vi "Set First Values.vi"(6 "PAYLOAD":u32[](array[numeric])=[0, 0, 0, 0, 0, 0, 0, 0, 0, 0, 0, 0, 0, 0, 0, 0, 0, 0, 0, 0, 0, 0, 0, 0, 0, 0, 0, 0, 0, 0, 0, 0, 0, 0, 0, 0, 0, 0, 0, 0, 0, 0, 0, 0, 0, 0, 0, 0, 0, 0, 0, 0, 0, 0, 0, 0, 0, 0, 0, 0, 0, 0, 0, 0] format="%x", 7 "TYPE":T1 items=["CAN Data"=0, "CAN Remote"=1, "CAN Bus Error"=2, "CAN 2.0 Data"=8, "CAN FD Data"=16, "CAN FD+BRS Data"=24, "J1939 Data"=192, "Delay"=224, "Log Trigger"=225, "Start Trigger"=226], 8 "error":errorcluster, 9 "DLC":u32 format="%x", 10 "IDENTIFIER":u32 format="%x", 11 "gRPC ID In":T2) -> (0 "error out":errorcluster, 3 "gRPC ID Out":T2)   [LabVIEW 2025]
uses:
  <vilib>/gRPC/LabVIEW gRPC Library/Shared/grpcId.ctl
  OOB gRPC Client/RPC Messages/hwval_GenericRequest.ctl
  OOB gRPC Client/OOB gRPC Client.lvlib
  <vilib>/gRPC/LabVIEW gRPC Library/grpc-lvsupport-release.lvlib
  XNET Frame Type CAN.ctl
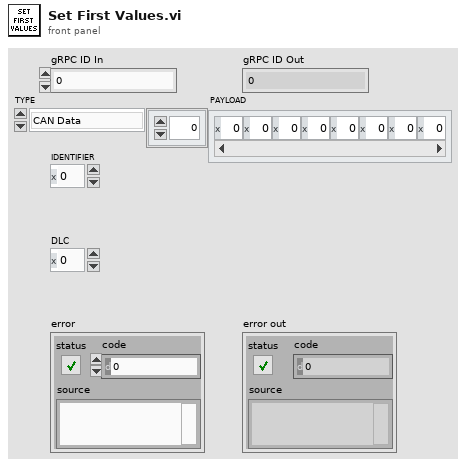
[diagram p1: front panel]
types:
  T1 = typedef "XNET Frame Type CAN.ctl" = u32
  T2 = typedef "grpc-lvsupport-release.lvlib/grpcId.ctl" = u64
  T3 = typedef "OOB gRPC Client.lvlib/hwval_GenericRequest.ctl" = cluster{"Command":string, "Payload":u8[]}
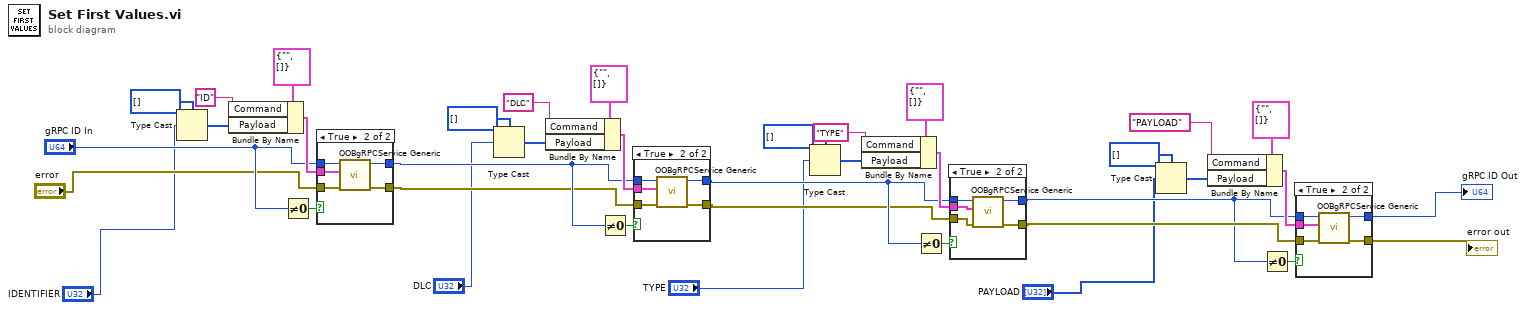
[diagram p0: block diagram]
diagram:
  n1 = Type Cast(type=u8[] [] ("Payload"), x="IDENTIFIER") -> (*(type *) &x=w35:u8[])
  n2 = Bundle By Name(cluster=T3 {"Command"="", "Payload"=[]} ("hwval_GenericRequest"), "Command"="ID", "Payload"=w35) -> (w34:T3)
  n3 = Not Equal To 0?(x="gRPC ID In") -> (x != 0?=w33:bool)
  n4 = case shown="True" w33 {
    tunnel: [w40 w42] -> w23
    tunnel: [w39 w41] -> w22
    tunnel: "gRPC ID In" -> [w40 w45]
    tunnel: "error" -> [w39 w44]
    tunnel: w34 -> [_ w43]
    frame False {
    }
    frame True {
      n5 = call "OOBgRPCService Generic.vi"("error in"=w44, "Request Data"=w43, "gRPC ID"=w45) -> ("error out"=w41:errorcluster, "gRPC ID out"=w42:T2)  [unwired: 6 in, 1 out]
    }
  }
  n6 = Type Cast(type=u8[] [] ("Payload"), x="DLC") -> (*(type *) &x=w26:u8[])
  n7 = Bundle By Name(cluster=T3 {"Command"="", "Payload"=[]} ("hwval_GenericRequest"), "Command"="DLC", "Payload"=w26) -> (w25:T3)
  n8 = Not Equal To 0?(x=w23) -> (x != 0?=w24:bool)
  n9 = case shown="True" w24 {
    tunnel: [w47 w49] -> w14
    tunnel: [w46 w48] -> w13
    tunnel: w23 -> [w47 w52]
    tunnel: w22 -> [w46 w51]
    tunnel: w25 -> [_ w50]
    frame False {
    }
    frame True {
      n10 = call "OOBgRPCService Generic.vi"("error in"=w51, "Request Data"=w50, "gRPC ID"=w52) -> ("error out"=w48:errorcluster, "gRPC ID out"=w49:T2)  [unwired: 6 in, 1 out]
    }
  }
  n11 = Type Cast(type=u8[] [] ("Payload"), x="TYPE") -> (*(type *) &x=w17:u8[])
  n12 = Bundle By Name(cluster=T3 {"Command"="", "Payload"=[]} ("hwval_GenericRequest"), "Command"="TYPE", "Payload"=w17) -> (w16:T3)
  n13 = Not Equal To 0?(x=w14) -> (x != 0?=w15:bool)
  n14 = case shown="True" w15 {
    tunnel: [w54 w56] -> w4
    tunnel: [w53 w55] -> w5
    tunnel: w14 -> [w54 w59]
    tunnel: w13 -> [w53 w58]
    tunnel: w16 -> [_ w57]
    frame False {
    }
    frame True {
      n15 = call "OOBgRPCService Generic.vi"("error in"=w58, "Request Data"=w57, "gRPC ID"=w59) -> ("error out"=w55:errorcluster, "gRPC ID out"=w56:T2)  [unwired: 6 in, 1 out]
    }
  }
  n16 = Type Cast(type=u8[] [] ("Payload"), x="PAYLOAD") -> (*(type *) &x=w8:u8[])
  n17 = Bundle By Name(cluster=T3 {"Command"="", "Payload"=[]} ("hwval_GenericRequest"), "Command"="PAYLOAD", "Payload"=w8) -> (w7:T3)
  n18 = Not Equal To 0?(x=w4) -> (x != 0?=w6:bool)
  n19 = case shown="True" w6 {
    tunnel: [w61 w63] -> w1
    tunnel: [w60 w62] -> w2
    tunnel: w4 -> [w61 w66]
    tunnel: w5 -> [w60 w65]
    tunnel: w7 -> [_ w64]
    frame False {
    }
    frame True {
      n20 = call "OOBgRPCService Generic.vi"("error in"=w65, "Request Data"=w64, "gRPC ID"=w66) -> ("error out"=w62:errorcluster, "gRPC ID out"=w63:T2)  [unwired: 6 in, 1 out]
    }
  }
  "error out" <- w2
  "gRPC ID Out" <- w1
